vi "Drive SSI.vi"(10 "Drive SS State":T2, 11 "Robot Controls":T3) -> (3 "Drive SS Actuator Values Out":T1)   [LabVIEW 2014]
uses:
  Robot Commands.ctl
  Drive SS State.ctl
  Drive SS Actuator Values.ctl
  <vilib>/Rock Robotics/WPI/DriverStation/WPI_DriverStationRobotMode2.ctl
  Robot Global Data.vi
  Global Variables/Refnum Names.vi
  Global Variables/Settings.vi
panel:
  # "Field Centric"
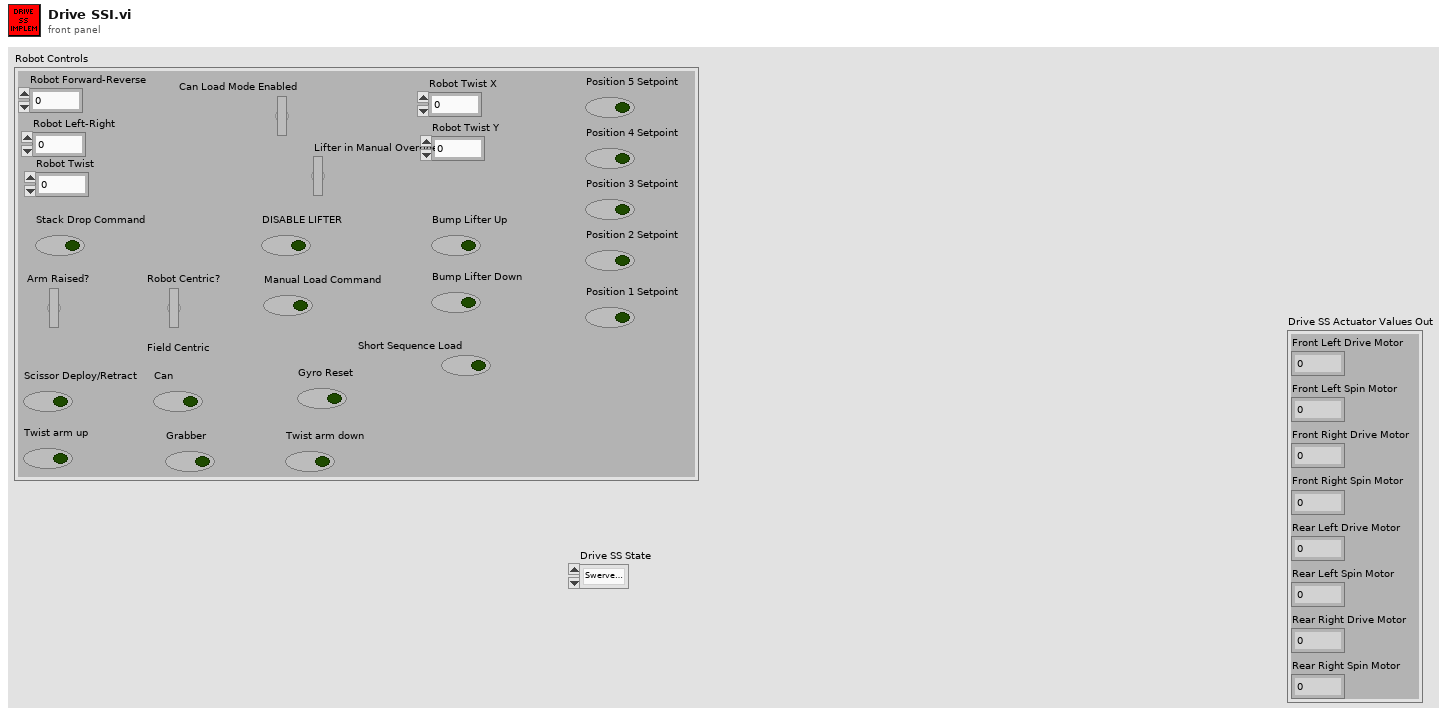
[diagram p1: front panel]
types:
  T1 = typedef "Drive SS Actuator Values.ctl" = cluster{"Front Left Drive Motor":dbl, "Front Left Spin Motor":dbl, "Front Right Drive Motor":dbl, "Front Right Spin Motor":dbl, "Rear Left Drive Motor":dbl, "Rear Left Spin Motor":dbl, "Rear Right Drive Motor":dbl, "Rear Right Spin Motor":dbl}
  T2 = typedef "Drive SS State.ctl" = enum16{"Swerve Drive", "Arcade Drive", "Mecanum Drive"}
  T3 = typedef "Robot Commands.ctl" = cluster{"Robot Forward-Reverse":dbl, "Robot Left-Right":dbl, "Robot Twist":dbl, "Can Load Mode Enabled":bool, "Lifter in Manual Override?":bool, "Stack Drop Command":bool, "Arm Raised?":bool, "DISABLE LIFTER":bool, "Position 1 Setpoint":bool, "Position 2 Setpoint":bool, "Position 3 Setpoint":bool, "Position 4 Setpoint":bool, "Position 5 Setpoint":bool, "Bump Lifter Down":bool, "Bump Lifter Up":bool, "Manual Load Command":bool, "Robot Centric?":bool, "Scissor Deploy/Retract":bool, "Grabber":bool, "Can":bool, "Twist arm up":bool, "Gyro Reset":bool, "Twist arm down":bool, "Short Sequence Load":bool, "Robot Twist X":dbl, "Robot Twist Y":dbl}
  T4 = typedef "WPI_DriverStationRobotMode2.ctl" = enum16{"Autonomous Disabled", "Autonomous Enabled", "Teleop Disabled", "Teleop Enabled", "Disconnected", "Finish", "Test Disabled", "Test Enabled", "Emergency Stopped"}
  T5 = typedef "WPI_GyroDevRef.ctl" = cluster{"DevStatus":errorcluster, "Analog Module":T6, "Analog Channel":T7, "Offset":dbl, "Gain (VoltsPerDegree/Second)":dbl}
  T6 = typedef "FPGA_TypedefAnalogModule.ctl" = enum16{"Controller 1"}
  T7 = typedef "FPGA_AIChannel.ctl" = enum8{"AI 0", "AI 1", "AI 2", "AI 3", "AI MXP 0", "AI MXP 1", "AI MXP 2", "AI MXP 3", "Invalid"}
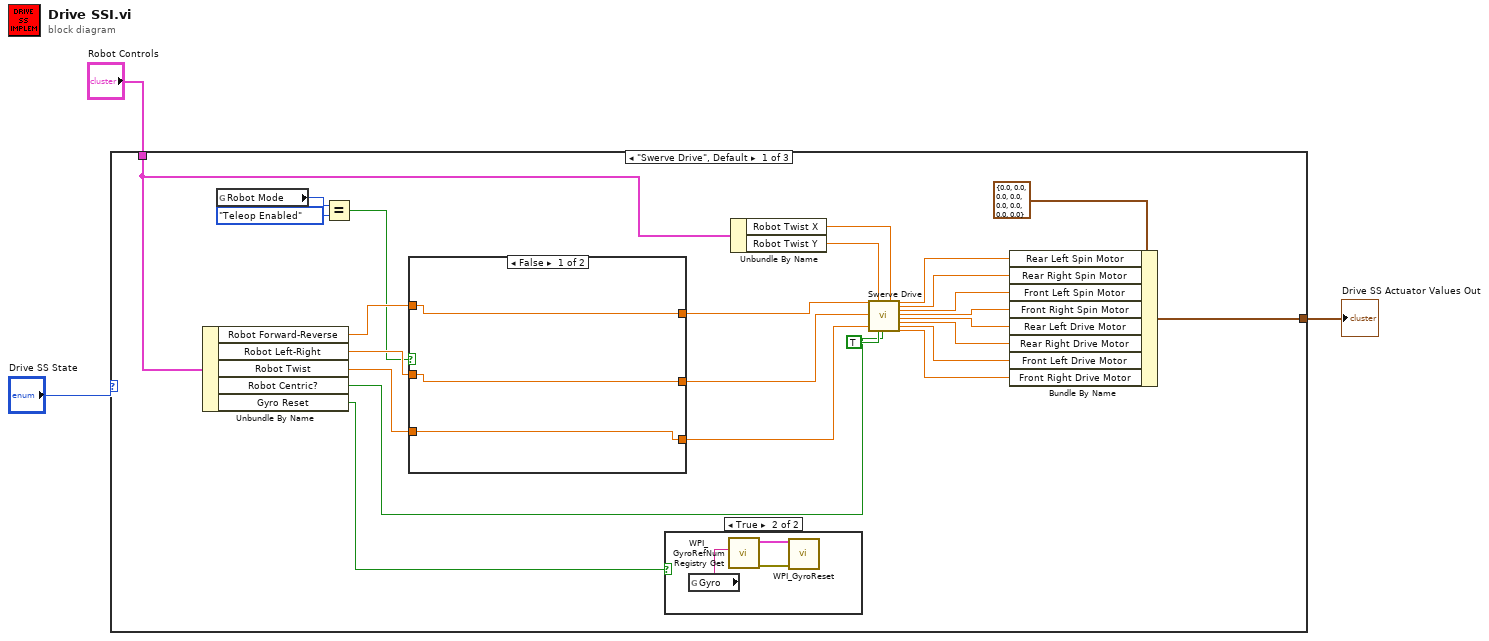
[diagram p0: block diagram]
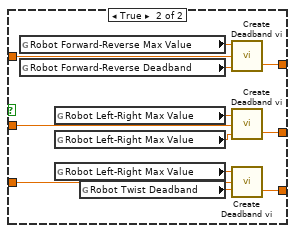
[diagram p2: hidden frame]
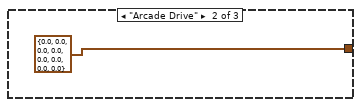
[diagram p4: hidden frame]
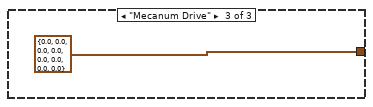
[diagram p5: hidden frame]
diagram:
  n1 = case shown="\"Swerve Drive\", Default" "Drive SS State" {
    tunnel: "Robot Controls" -> [w6 _ _]
    tunnel: [w26 T1 {"Front Left Drive Motor"=0.0, "Front Left Spin Motor"=0.0, "Front Right Drive Motor"=0.0, "Front Right Spin Motor"=0.0, "Rear Left Drive Motor"=0.0, "Rear Left Spin Motor"=0.0, "Rear Right Drive Motor"=0.0, "Rear Right Spin Motor"=0.0} ("Drive SS Actuator Values Out 2") T1 {"Front Left Drive Motor"=0.0, "Front Left Spin Motor"=0.0, "Front Right Drive Motor"=0.0, "Front Right Spin Motor"=0.0, "Rear Left Drive Motor"=0.0, "Rear Left Spin Motor"=0.0, "Rear Right Drive Motor"=0.0, "Rear Right Spin Motor"=0.0} ("Drive SS Actuator Values Out 2")] -> w1
    frame "Swerve Drive", Default {
      n2 = Unbundle By Name(w6) -> ("Robot Forward-Reverse"=w12:dbl, "Robot Left-Right"=w14:dbl, "Robot Twist"=w16:dbl, "Robot Centric?"=w11:bool, "Gyro Reset"=w10:bool)
      n3 = global read "Robot Global Data.vi" "Robot Mode"() -> (w9:T4)
      n4 = Equal?(x=w9, y=WPI_DriverStationRobotMode2."Teleop Enabled") -> (x = y?=w7:bool)
      n5 = case shown="False" w7 {
        tunnel: [w29 w43] -> w17
        tunnel: w16 -> [w29 w42]
        tunnel: [w30 w41] -> w15
        tunnel: w14 -> [w30 w40]
        tunnel: [w31 w39] -> w13
        tunnel: w12 -> [w31 w38]
        frame False {
        }
        frame True {
          n6 = global read "Settings.vi" "Robot Forward-Reverse Max Value"() -> (w37:dbl)
          n7 = global read "Settings.vi" "Robot Forward-Reverse Deadband"() -> (w36:dbl)
          n8 = global read "Settings.vi" "Robot Left-Right Max Value"() -> (w35:dbl)
          n9 = global read "Settings.vi" "Robot Left-Right Max Value"() -> (w34:dbl)
          n10 = global read "Settings.vi" "Robot Left-Right Max Value"() -> (w33:dbl)
          n11 = global read "Settings.vi" "Robot Twist Deadband"() -> (w32:dbl)
          n12 = call "Create Deadband vi.vi"("Input Deadband"=w36, "Input"=w38, "Output Upper Limit"=w37) -> ("Output"=w39:dbl)  [unwired: 1 in]
          n13 = call "Create Deadband vi.vi"("Input Deadband"=w34, "Input"=w40, "Output Upper Limit"=w35) -> ("Output"=w41:dbl)  [unwired: 1 in]
          n14 = call "Create Deadband vi.vi"("Input Deadband"=w32, "Input"=w42, "Output Upper Limit"=w33) -> ("Output"=w43:dbl)  [unwired: 1 in]
        }
      }
      n15 = case shown="True" w10 {
        frame False {
        }
        frame True {
          n16 = global read "Refnum Names.vi" "Gyro"() -> (w44:string)
          n17 = call <vilib>:"WPI_GyroRefNum Registry Get.vi"("refnum name"=w44) -> ("error out"=w45:errorcluster, "GyroDevRef"=w46:T5)  [unwired: 9 in]
          n18 = call <vilib>:"WPI_GyroReset.vi"("error in (no error)"=w45, "GyroDevRef"=w46) -> ()  [unwired: 8 in, 2 out]
        }
      }
      n19 = Unbundle By Name(w6) -> ("Robot Twist X"=w5:dbl, "Robot Twist Y"=w4:dbl)
      n20 = call "Swerve Drive.vi"("X"=w13, "Y"=w15, "Z"=w17, "Rot. Point Y"=w4, "Auto Controls"=TRUE, "Robot-Centric"=w11, "Rot. Point X"=w5) -> ("Back left Spin Power"=w25:dbl, "Back Right Spin Power"=w24:dbl, "Front left Spin Power"=w23:dbl, "Front Right Spin Power"=w22:dbl, "Back left Motor Power"=w21:dbl, "Back Right Motor Power"=w20:dbl, "Front left Motor Power"=w19:dbl, "Front Right Motor Power"=w18:dbl)  [unwired: 13 in]
      n21 = Bundle By Name(cluster=T1 {"Front Left Drive Motor"=0.0, "Front Left Spin Motor"=0.0, "Front Right Drive Motor"=0.0, "Front Right Spin Motor"=0.0, "Rear Left Drive Motor"=0.0, "Rear Left Spin Motor"=0.0, "Rear Right Drive Motor"=0.0, "Rear Right Spin Motor"=0.0} ("Drive SS Actuator Values Out 2"), "Rear Left Spin Motor"=w25, "Rear Right Spin Motor"=w24, "Front Left Spin Motor"=w23, "Front Right Spin Motor"=w22, "Rear Left Drive Motor"=w21, "Rear Right Drive Motor"=w20, "Front Left Drive Motor"=w19, "Front Right Drive Motor"=w18) -> (w26:T1)
    }
    frame "Arcade Drive" {
    }
    frame "Mecanum Drive" {
    }
  }
  "Drive SS Actuator Values Out" <- w1
